vi "Hexa to Long.vi"(0 "Hexa":string, 1 "Index":i32) -> (5 "Long":u32)   [LabVIEW 2017]
doc: "Long aus Trackerantwort (Hexa)\n\nIndex: \n0 = Size\n4 = Datatype\n8 = Command \n12 = Result Status"
panel:
  # "Index: \n0 = Länge Befehl\n4 = Datatype\n8 = Command\n12 = Result Status"
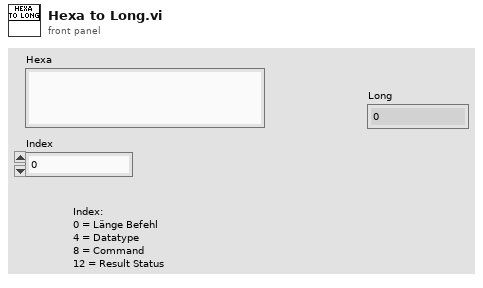
[diagram p1: front panel]
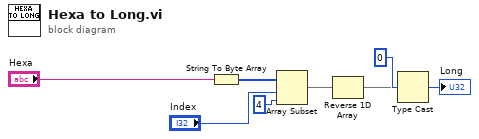
[diagram p0: block diagram]
diagram:
  n1 = String To Byte Array(string="Hexa") -> (unsigned byte array=w8:u8[])
  n2 = Array Subset(array=w8, index="Index", length=4 ("Länge")) -> (w6:u8[])
  n3 = Reverse 1D Array(array=w6) -> (reversed array=w5:u8[])
  n4 = Type Cast(type=0, x=w5) -> (*(type *) &x=→"Long":i32)
